vi "LM Asymmetric Gaussian and gradient.vi"(3 "output control":T1, 4 "data":variant, 5 "X":dbl[](array[numeric]), 6 "a":dbl[](array[numeric])) -> (0 "error out":errorcluster, 1 "f'(X,a)":dbl[][](array[numeric]), 2 "f(X,a)":dbl[](array[numeric]))   [LabVIEW 2021, in "Fits.lvlib"]
doc: "This template is the starting point for creating a model function to be passed to the Nonlinear Curve Fit.vi."
uses:
  Fits.lvlib
  <vilib>/gmath/NumericalOptimization/LM_output select.ctl
  <vilib>/gmath/NI_Gmath.lvlib
panel:
  # "Parameters:\n\namplitude: A\ncenter: t_0\nSDV-: s-\nSDV+: s+"
  # "see the License on the block diagram (Ctrl+E or Window:Show Block Diagram)"
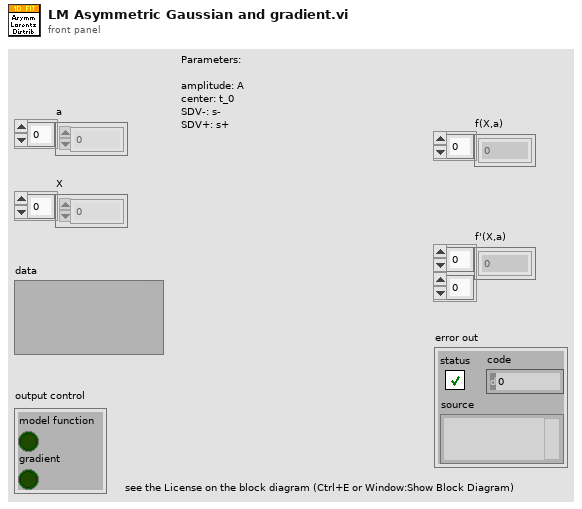
[diagram p1: front panel]
types:
  T1 = typedef "NI_Gmath.lvlib/LM_output select.ctl" = cluster{"model function":bool, "gradient":bool}
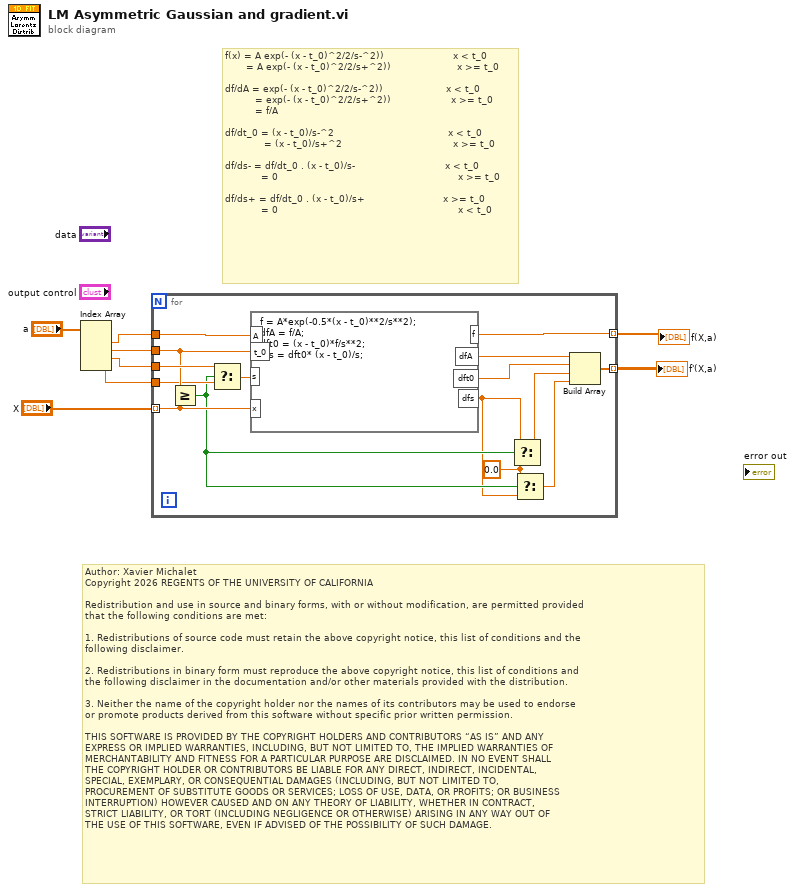
[diagram p0: block diagram]
diagram:
  # "Author: Xavier Michalet\nCopyright 2026 REGENTS OF THE UNIVERSITY OF CALIFORNIA\n\nRedistribution and use in source and binary forms, with or without modification, are permitted provided\nthat the following conditions are met:\n\n1. Redistributions of source code must retain the above copyright notice, this list of conditions and the\nfollowing disclaimer.\n\n2. Redistributions in binary form must reproduce the above copyright notice, this list of conditions and\nthe following disclaimer in the documentation and/or other materials provided with the distribution.\n\n3. Neither the name of the copyright holder nor the names of its contributors may be used to endorse \nor promote products derived from this software without specific prior written permission.\n\nTHIS SOFTWARE IS PROVIDED BY THE COPYRIGHT HOLDERS AND CONTRIBUTORS “AS IS” AND ANY \nEXPRESS OR IMPLIED WARRANTIES, INCLUDING, BUT NOT LIMITED TO, THE IMPLIED WARRANTIES OF\nMERCHANTABILITY AND FITNESS FOR A PARTICULAR PURPOSE ARE DISCLAIMED. IN NO EVENT SHALL\nTHE COPYRIGHT HOLDER OR CONTRIBUTORS BE LIABLE FOR ANY DIRECT, INDIRECT, INCIDENTAL, \nSPECIAL, EXEMPLARY, OR CONSEQUENTIAL DAMAGES (INCLUDING, BUT NOT LIMITED TO, \nPROCUREMENT OF SUBSTITUTE GOODS OR SERVICES; LOSS OF USE, DATA, OR PROFITS; OR BUSINESS\nINTERRUPTION) HOWEVER CAUSED AND ON ANY THEORY OF LIABILITY, WHETHER IN CONTRACT, \nSTRICT LIABILITY, OR TORT (INCLUDING NEGLIGENCE OR OTHERWISE) ARISING IN ANY WAY OUT OF\nTHE USE OF THIS SOFTWARE, EVEN IF ADVISED OF THE POSSIBILITY OF SUCH DAMAGE."
  # "f(x) = A exp(- (x - t_0)^2/2/s-^2))                       x < t_0\n       = A exp(- (x - t_0)^2/2/s+^2))                      x >= t_0\n\ndf/dA = exp(- (x - t_0)^2/2/s-^2))                     x < t_0\n          = exp(- (x - t_0)^2/2/s+^2))                    x >= t_0\n          = f/A\n\ndf/dt_0 = (x - t_0)/s-^2                                      x < t_0\n             = (x - t_0)/s+^2                                     x >= t_0\n\ndf/ds- = df/dt_0 . (x - t_0)/s-                              x < t_0\n            = 0                                                            x >= t_0\n\ndf/ds+ = df/dt_0 . (x - t_0)/s+                          x >= t_0\n            = 0                                                            x < t_0"
  n1 = Index Array(array="a") -> (element #1=w7:dbl, element #2=w6:dbl, element #3=w5:dbl, element #4=w4:dbl)  [unwired: 4 in]
  n2 = for {
    tunnel: w7 -> [w23]
    tunnel: w6 -> [w20]
    tunnel: w5 -> [w22]
    tunnel: w4 -> [w18]
    tunnel: "X" -> [w19] mode=indexing
    tunnel: [w13] -> w2 mode=indexing
    tunnel: [w9] -> w1 mode=indexing
    w16 = 0.0 ("f")
    n3 = Greater Or Equal?(x=w20, y=w19) -> (x >= y?=w17:bool)
    n4 = Select(t=w22, s=w17, f=w18) -> (s? t:f=w21:dbl)
    n5 = formula code="f = A*exp(-0.5*(x - t_0)**2/s**2);\ndfA = f/A;\ndft0 = (x - t_0)*f/s**2;\ndfs = dft0* (x - t_0)/s;"("A"=w23, "t_0"=w20, "s"=w21, "x"=w19) -> ("f"=w13:dbl, "dfA"=w14:dbl, "dft0"=w12:dbl, "dfs"=w15:dbl)
    n6 = Select(t=w15, s=w17, f=w16) -> (s? t:f=w11:dbl)
    n7 = Select(t=w16, s=w17, f=w15) -> (s? t:f=w10:dbl)
    n8 = Build Array(w14, w12, w11, w10) -> (w9:dbl[])
  }
  "f(X,a)" <- w2
  "f'(X,a)" <- w1
